vi "2023_day04 Recursive Search (SubVI).vi"(8 "Number of Cards In":i32, 9 "Top Level-Index In":i32, 10 "All Scratchcards":string[](array[string])) -> (0 "Number of Cards Out":i32, 1 "Top Level-Index Out":i32)   [LabVIEW 2021]
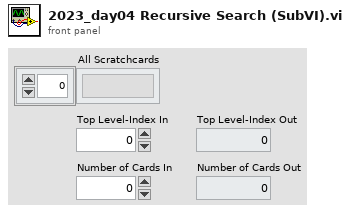
[diagram p1: front panel]
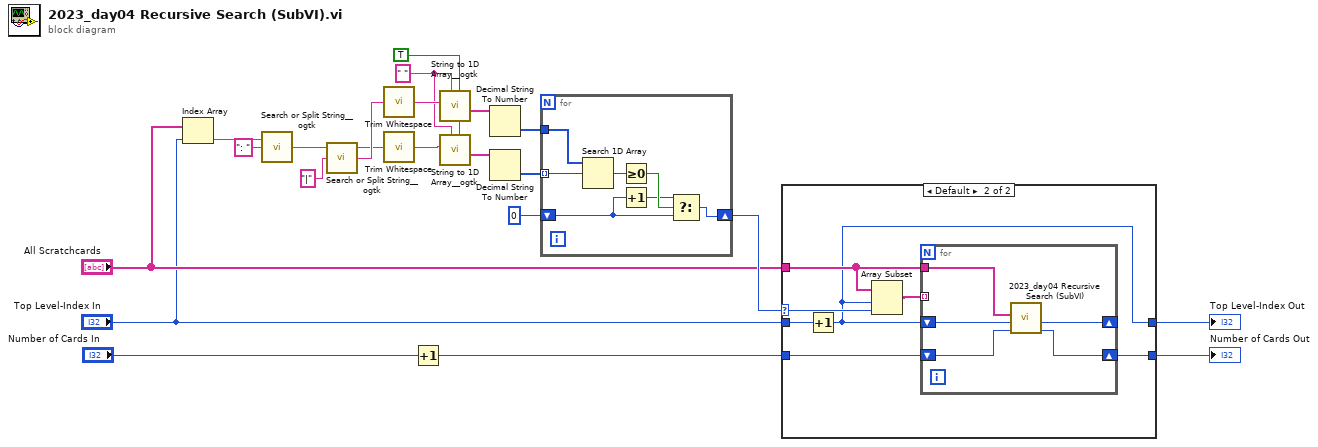
[diagram p0: block diagram]
diagram:
  w15 = TRUE ("ignore duplicate delimiters? (F=No)")
  w13 = " " ("delimiter (Tab)")
  n1 = Index Array(array="All Scratchcards", index="Top Level-Index In") -> (element=w6:string)
  n2 = call <userlib>:"Search or Split String__ogtk.vi"("search string/char (-)"=": ", "string"=w6) -> ("substring after match"=w10:string)  [unwired: 1 in, 2 out]
  n3 = call <userlib>:"Search or Split String__ogtk.vi"("search string/char (-)"="|", "string"=w10) -> ("substring after match"=w14:string, "substring before match"=w12:string)  [unwired: 1 in, 1 out]
  n4 = call <vilib>:"Trim Whitespace.vi"("string"=w14) -> ("trimmed string"=w21:string)  [unwired: 1 in]
  n5 = call <vilib>:"Trim Whitespace.vi"("string"=w12) -> ("trimmed string"=w22:string)  [unwired: 1 in]
  n6 = Increment(x="Number of Cards In") -> (x+1=w1:i32)
  n7 = call <userlib>:"String to 1D Array__ogtk.vi"("ignore duplicate delimiters? (F=No)"=w15, "delimiter (Tab)"=w13, "string"=w21) -> ("Array of Strings"=w17:string[])  [unwired: 8 in]
  n8 = call <userlib>:"String to 1D Array__ogtk.vi"("ignore duplicate delimiters? (F=No)"=w15, "delimiter (Tab)"=w13, "string"=w22) -> ("Array of Strings"=w16:string[])  [unwired: 8 in]
  n9 = Decimal String To Number(string=w17) -> (number=w20:i32[])  [unwired: 2 in, 1 out]
  n10 = Decimal String To Number(string=w16) -> (number=w18:i32[])  [unwired: 2 in, 1 out]
  n11 = for {
    tunnel: w18 -> [w28] mode=indexing
    tunnel: w20 -> [w29]
    shift-right: [w25] -> w8
    shift-left: 0 -> [w24]
    n12 = Search 1D Array(1D array=w29, element=w28) -> (index of element=w27:i32)  [unwired: 1 in]
    n13 = Greater Or Equal To 0?(x=w27) -> (x >= 0?=w26:bool)
    n14 = Increment(x=w24) -> (x+1=w23:i32)
    n15 = Select(t=w23, s=w26, f=w24) -> (s? t:f=w25:i32)
  }
  n16 = case shown="Default" w8 {
    selector: w8 -> [_ w34]
    tunnel: "All Scratchcards" -> [_ w38]
    tunnel: "Top Level-Index In" -> [w31 w33]
    tunnel: w1 -> [w30 w36]
    tunnel: [w30 w37] -> w3
    tunnel: [w31 w32] -> w4
    frame 0 {
    }
    frame Default {
      n17 = Increment(x=w33) -> (x+1=w32:i32)
      n18 = Array Subset(array=w38, index=w32, length=w34) -> (w35:string[])
      n19 = for {
        tunnel: w35 -> [_] mode=indexing
        tunnel: w38 -> [w43]
        shift-right: [w41] -> w37
        shift-left: w36 -> [w42]
        shift-right: [w39] -> _
        shift-left: w32 -> [w40]
        n20 = call "2023_day04 Recursive Search (SubVI).vi"("Number of Cards In"=w42, "Top Level-Index In"=w40, "All Scratchcards"=w43) -> ("Number of Cards Out"=w41:i32, "Top Level-Index Out"=w39:i32)  [unwired: 7 in]
      }
    }
  }
  "Number of Cards Out" <- w3
  "Top Level-Index Out" <- w4
